vi "DAQ Viewer-Core_Process.vi"(0 "FTW Actor Instance Configuration":string="{\n  \"Identity\": \"ActorName\",\n  \"InboxAddress\": \"inproc://*\",\n  \"PublisherAddress\": \"\",\n  \"LoggerAddress\": \"\",\n  \"DebugEnableInboxLogging\": false,\n  \"DebugEnableJobLogging\": false,\n  \"LauncherAddress\": \"\",\n  \"My Data\": false\n}", 11 "ErrorIn":errorcluster) -> (15 "Error":errorcluster)   [LabVIEW 2013, in "DAQ Viewer-Core.lvclass"]
uses:
  DAQ Viewer-Core.lvclass
  source/actor/Message/Base/FTW-Message.lvclass
  source/actor/Instance/FTW-ActorInstance.lvclass/FTW-ActorInstance.ctl
  source/actor/JobSequencer/FTW-SEQ-Current.vi
  source/actor/Instance/FTW-ActorInstance.lvclass
  source/actor/Message/Request/FTW-Message-IncomingRequest.lvclass
panel:
  # "#TODO\nhide controls for a GUI"
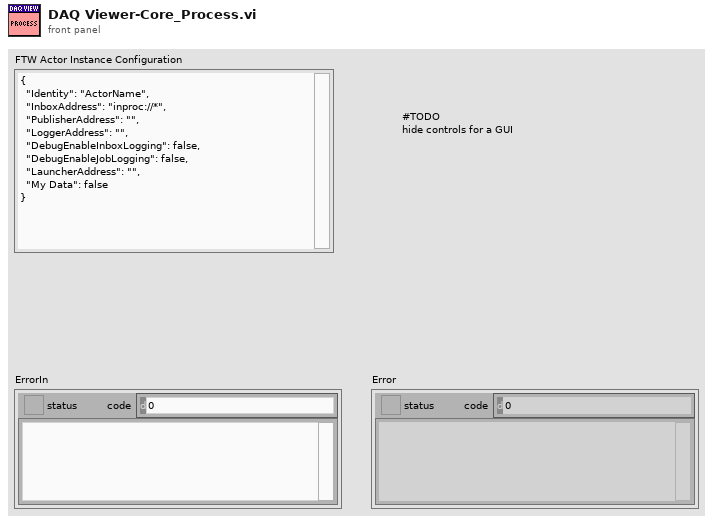
[diagram p1: front panel]
types:
  T1 = cluster{"Incoming Requests":refnum<event-registration>, "Local Messages":refnum<event-registration>, "Additional Registration Types":refnum<event-registration>}
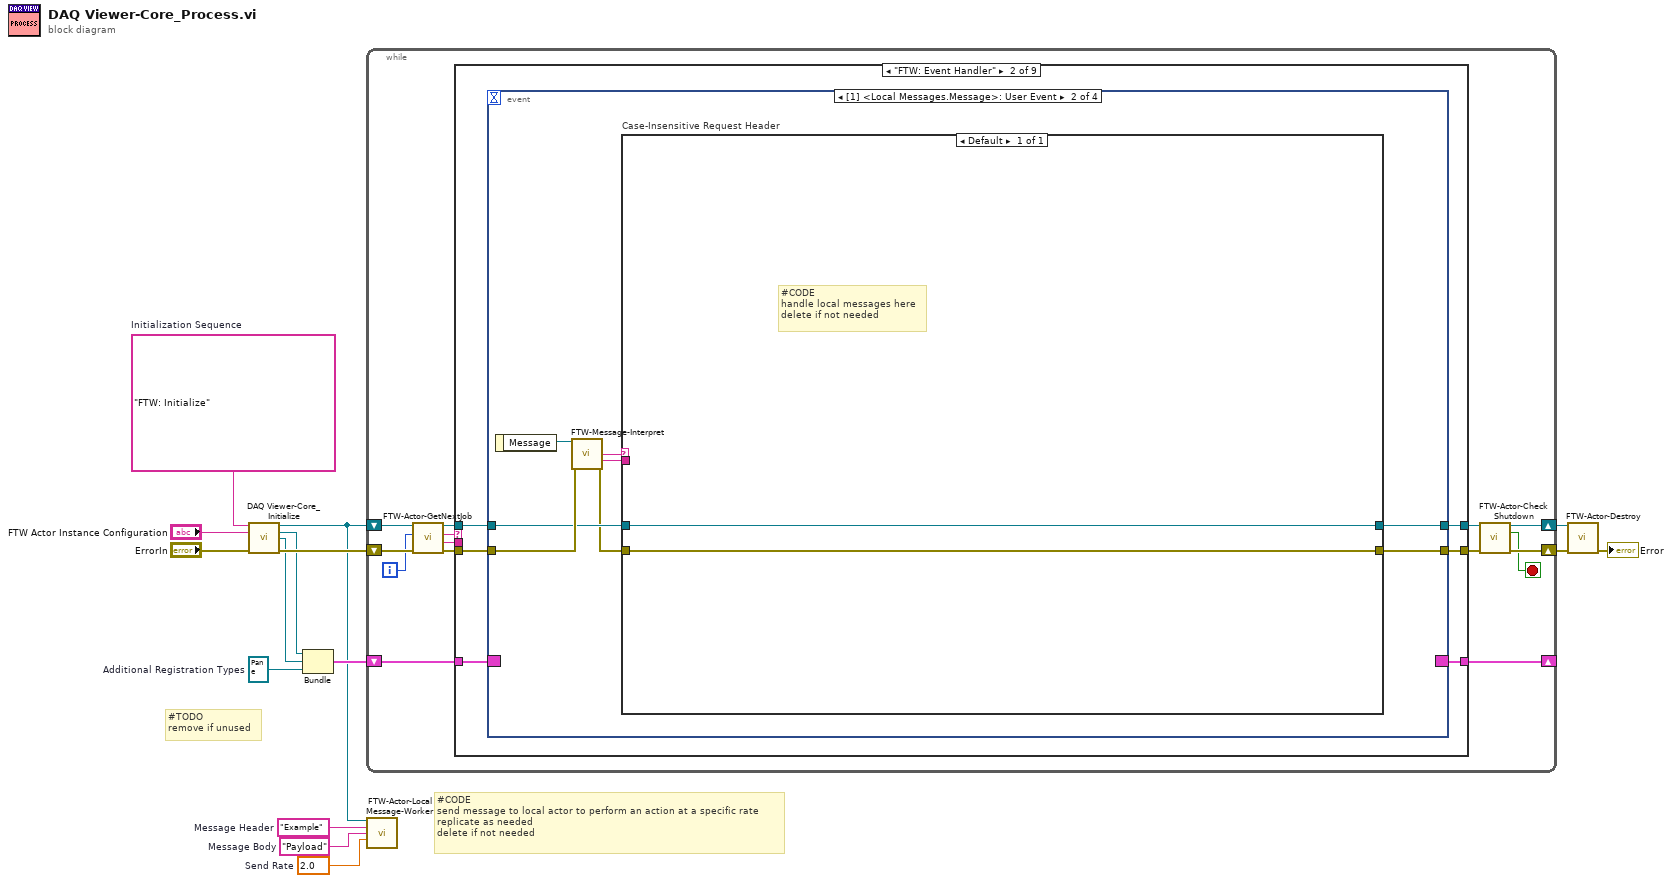
[diagram p0: block diagram]
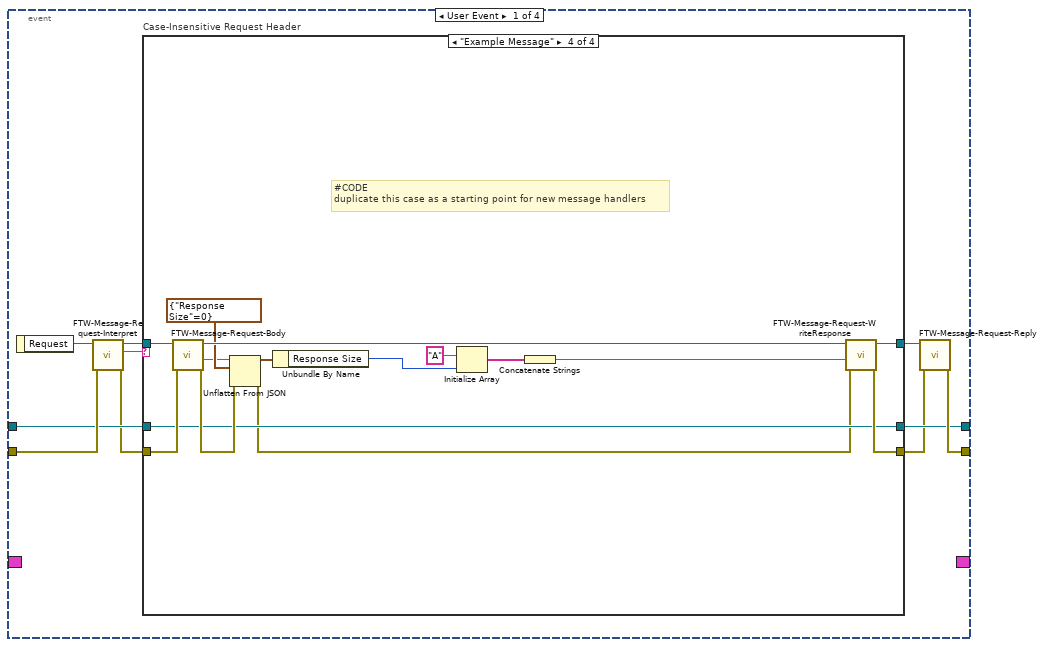
[diagram p3: hidden frame]
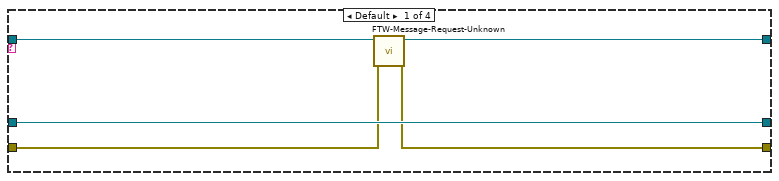
[diagram p4: hidden frame]
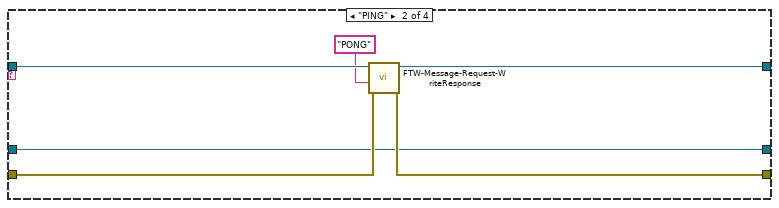
[diagram p5: hidden frame]
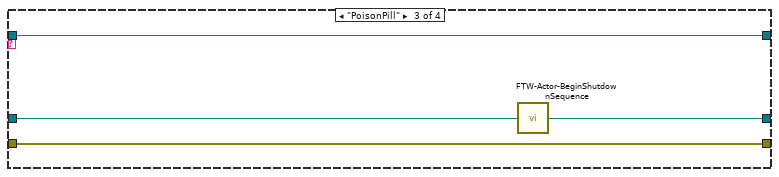
[diagram p6: hidden frame]
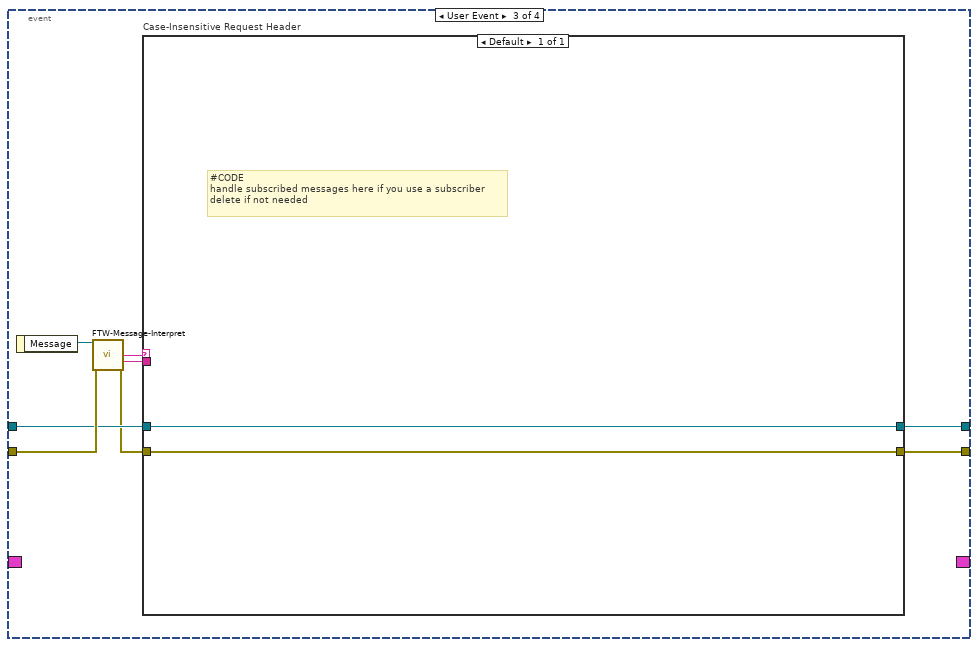
[diagram p7: hidden frame]
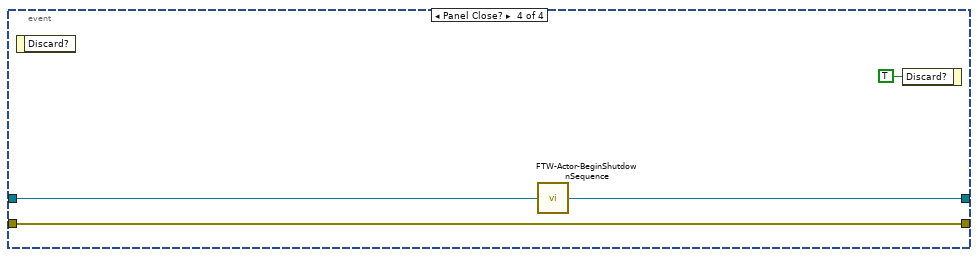
[diagram p8: hidden frame]
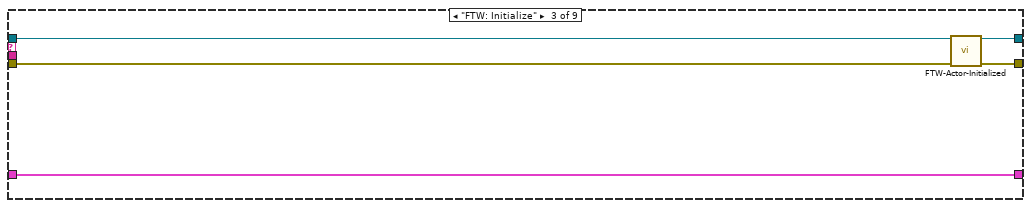
[diagram p9: hidden frame]
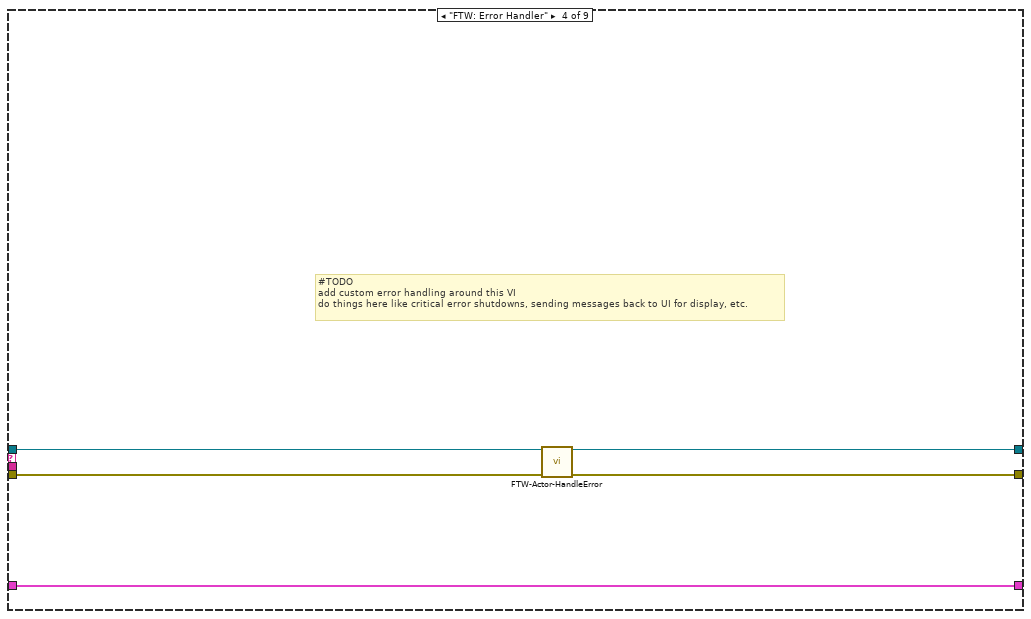
[diagram p10: hidden frame]
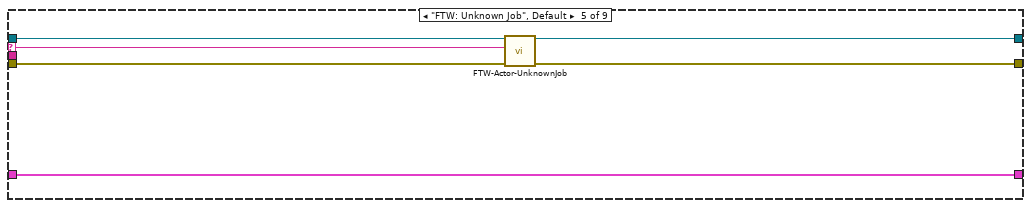
[diagram p11: hidden frame]
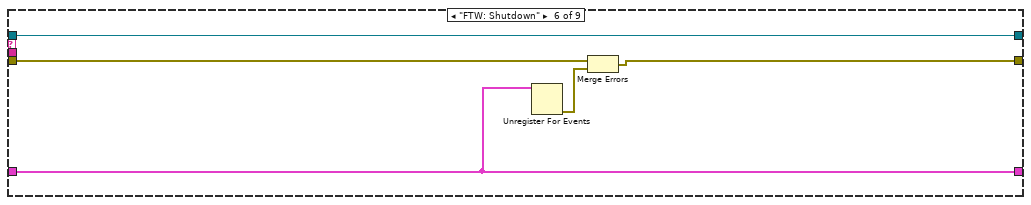
[diagram p12: hidden frame]
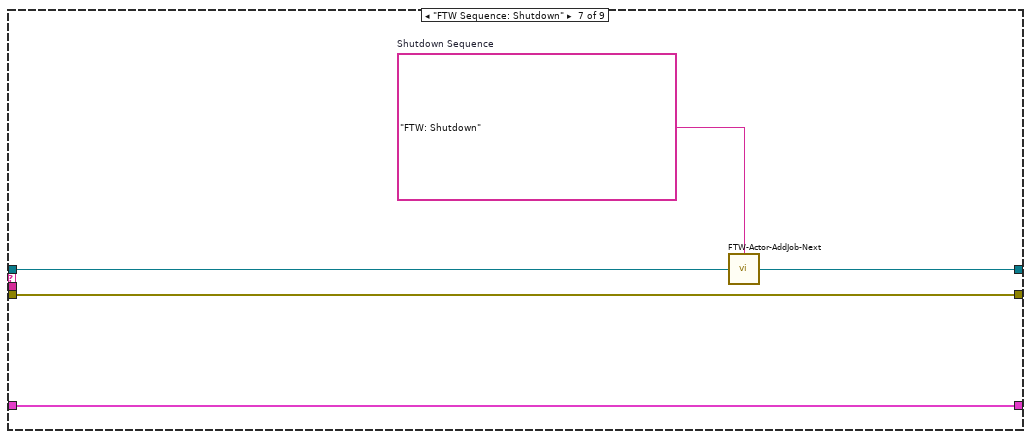
[diagram p13: hidden frame]
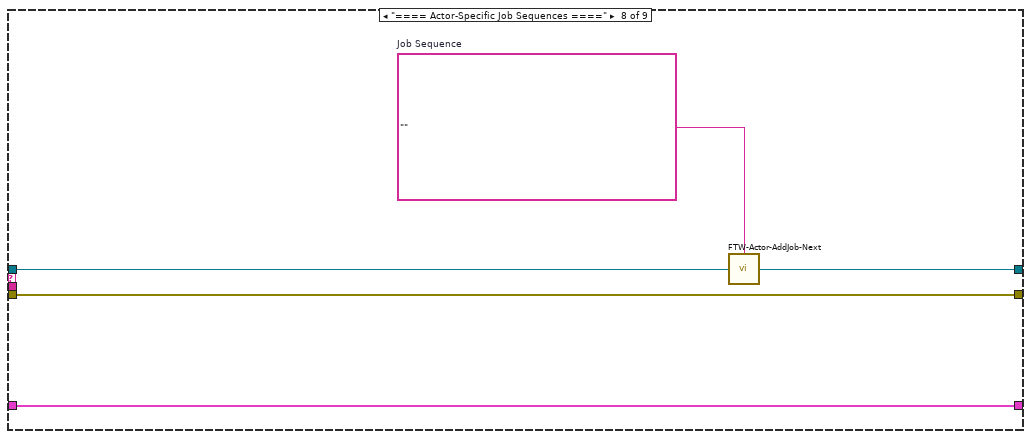
[diagram p14: hidden frame]
diagram:
  w2 = 2.0  # Send Rate
  w3 = "Payload"  # Message Body
  w4 = "Example"  # Message Header
  w5 = refnum<event-registration> refnum  # Additional Registration Types
  w11 = "FTW: Initialize"  # Initialization Sequence
  # "#CODE\nsend message to local actor to perform an action at a specific rate\nreplicate as needed\ndelete if not needed"
  # "#TODO\nremove if unused"
  n1 = call "DAQ Viewer-Core_Initialize.vi"("Initialization Sequence"=w11, "FTW Actor Instance Configuration"="FTW Actor Instance Configuration", "error in (no error)"="ErrorIn") -> ("Actor Template-Core out"=w1:refnum<class "DAQ Viewer-Core.lvclass">, "Incoming Requests"=w7:refnum<event-registration>, "Local Messages"=w6:refnum<event-registration>, "error out"=w12:errorcluster)  [unwired: 9 in]
  n2 = Bundle("Incoming Requests"=w7, "Local Messages"=w6, "Additional Registration Types"=w5) -> (w9:T1)  [unwired: 1 in]
  n3 = while {
    shift-right: [w19] -> w14
    shift-left: w12 -> [w26]
    shift-right: [w16] -> _
    shift-left: w9 -> [w29]
    shift-right: [w21] -> w15
    shift-left: w1 -> [w28]
    i -> [w17]
    stop <- w18 stop-if-true
    n4 = call "FTW-Actor-GetNextJob.vi"("error in"=w26, "Jobs Performed"=w17, "FTW Actor Instance"=w28) -> ("error out"=w25:errorcluster, "Job Data"=w23:string, "Job Name"=w24:string, "FTW Actor Instance out"=w27:refnum<class "DAQ Viewer-Core.lvclass">)  [unwired: 5 in]
    n5 = case shown="\"FTW: Event Handler\"" w24 {
      selector: w24 -> [_ _ _ _ w113 _ _ _ _]
      tunnel: [w31 w38 w103 w108 w116 w122 w127 w132 w136] -> w20
      tunnel: w25 -> [w31 w37 w106 w110 w117 w123 w127 w132 w136]
      tunnel: w29 -> [w32 w33 w107 w112 w118 w119 w128 w133 w135]
      tunnel: [w32 w36 w107 w112 w118 w119 w128 w133 w135] -> w16
      tunnel: w23 -> [_ _ _ _ _ _ _ _ _]
      tunnel: [w30 w35 w104 w109 w114 w120 w125 w130 w134] -> w22
      tunnel: w27 -> [w30 w34 w105 w111 w115 w120 w126 w131 w134]
      frame "==== Featherweight Framework Jobs ====" {
      }
      frame "FTW: Event Handler" {
        n6 = event shown="[1] <Local Messages.Message>: User Event" {
          selector: w33 -> [_ _ _ _]
          dyn-events: [_ _ _ _] -> w36
          timeout: _ -> [_ _ _ _]
          tunnel: [w47 w81 w91 w101] -> w38
          tunnel: w37 -> [w46 w85 w95 w101]
          tunnel: [w41 w82 w92 w99] -> w35
          tunnel: w34 -> [w45 w84 w94 w100]
          event User Event {
            n7 = event-data() -> ("Request"=w48:refnum<class "FTW-Message-IncomingRequest.lvclass">)  [unwired: 1 in]
            n8 = call "FTW-Message-Request-Interpret.vi"("error in"=w46, "FTW Incoming Request"=w48) -> ("error out"=w44:errorcluster, "Request Header"=w42:string, "FTW Incoming Request out"=w43:refnum<class "FTW-Message-IncomingRequest.lvclass">)  [unwired: 5 in, 2 out]
            n9 = case "Case-Insensitive Request Header" shown="\"Example Message\"" w42 {
              tunnel: [w51 w57 w62 w75] -> w40
              tunnel: w44 -> [w52 w58 w62 w78]
              tunnel: [w53 w56 w63 w72] -> w41
              tunnel: w45 -> [w53 w56 w61 w72]
              tunnel: w43 -> [w50 w59 w60 w76]
              tunnel: [w49 w55 w60 w73] -> w39
              frame Default {
                n10 = call "FTW-Message-Request-Unknown.vi"("error in"=w52, "FTW Incoming Request"=w50) -> ("error out"=w51:errorcluster, "FTW Incoming Request Out"=w49:refnum<class "FTW-Message-IncomingRequest.lvclass">)  [unwired: 8 in]
              }
              frame "PING" {
                n11 = call "FTW-Message-Request-WriteResponse.vi"("error in"=w58, "Response Body"="PONG" ("Response Header"), "FTW Incoming Request"=w59) -> ("error out"=w57:errorcluster, "FTW Incoming Request out"=w55:refnum<class "FTW-Message-IncomingRequest.lvclass">)  [unwired: 7 in]
              }
              frame "PoisonPill" {
                n12 = call "FTW-Actor-BeginShutdownSequence.vi"("FTW Actor Instance"=w61) -> ("FTW Actor Instance out"=w63:refnum<class "DAQ Viewer-Core.lvclass">)  [unwired: 3 in]
              }
              frame "Example Message" {
                # "#CODE\nduplicate this case as a starting point for new message handlers"
                n13 = call "FTW-Message-Request-Body.vi"("error in"=w78, "FTW Incoming Request"=w76) -> ("error out"=w77:errorcluster, "Request Body"=w69:string, "FTW Incoming Request out"=w74:refnum<class "FTW-Message-IncomingRequest.lvclass">)  [unwired: 7 in]
                n14 = Unflatten From JSON(JSON string=w69, type and defaults=cluster{"Response Size":i32} {"Response Size"=0}, error in (no error)=w77) -> (value=w68:cluster{"Response Size":i32}, error out=w71:errorcluster)  [unwired: 4 in]
                n15 = Unbundle By Name(w68) -> ("Response Size"=w67:i32)
                n16 = Initialize Array("A", w67) -> (w65:string[])
                n17 = Concatenate Strings(w65) -> (w64:string)
                n18 = call "FTW-Message-Request-WriteResponse.vi"("error in"=w71, "Response Body"=w64, "FTW Incoming Request"=w74) -> ("error out"=w75:errorcluster, "FTW Incoming Request out"=w73:refnum<class "FTW-Message-IncomingRequest.lvclass">)  [unwired: 7 in]
              }
            }
            n19 = call "FTW-Message-Request-Reply.vi"("FTW: Reply Error"=w40, "FTW Incoming Request"=w39) -> ("error out"=w47:errorcluster)  [unwired: 8 in, 1 out]
          }
          event User Event {
            n20 = event-data() -> ("Message"=w86:refnum<class "FTW-Message.lvclass">)  [unwired: 1 in]
            n21 = call-dynamic "FTW-Message-Interpret.vi"("FTW Message"=w86, "error in"=w85) -> ("Message Header"=w80:string, "Message Body"=w79:string, "error out"=w83:errorcluster)  [unwired: 9 in, 2 out]
            n22 = case "Case-Insensitive Request Header" shown="Default" w80 {
              tunnel: [w87] -> w81
              tunnel: w83 -> [w87]
              tunnel: [w88] -> w82
              tunnel: w84 -> [w88]
              tunnel: w79 -> [_]
              frame Default {
                # "#CODE\nhandle local messages here\ndelete if not needed"
              }
            }
          }
          event User Event {
            n23 = event-data() -> ("Message"=w96:refnum<class "FTW-Message.lvclass">)  [unwired: 1 in]
            n24 = call-dynamic "FTW-Message-Interpret.vi"("FTW Message"=w96, "error in"=w95) -> ("Message Header"=w90:string, "Message Body"=w89:string, "error out"=w93:errorcluster)  [unwired: 9 in, 2 out]
            n25 = case "Case-Insensitive Request Header" shown="Default" w90 {
              tunnel: [w97] -> w91
              tunnel: w93 -> [w97]
              tunnel: [w98] -> w92
              tunnel: w94 -> [w98]
              tunnel: w89 -> [_]
              frame Default {
                # "#CODE\nhandle subscribed messages here if you use a subscriber\ndelete if not needed"
              }
            }
          }
          event Panel Close? {
            n26 = event-data() -> ()  [unwired: 1 in, 1 out]
            n27 = call "FTW-Actor-BeginShutdownSequence.vi"("FTW Actor Instance"=w100) -> ("FTW Actor Instance out"=w99:refnum<class "DAQ Viewer-Core.lvclass">)  [unwired: 3 in]
            n28 = event-data("Discard?"=TRUE) -> ()  [unwired: 1 in, 1 out]
          }
        }
      }
      frame "FTW: Initialize" {
        n29 = call-dynamic "FTW-Actor-Initialized.vi"("FTW Actor Instance"=w105, "error in"=w106) -> ("FTW Actor Instance out"=w104:refnum<class "DAQ Viewer-Core.lvclass">, "error out"=w103:errorcluster)  [unwired: 12 in]
      }
      frame "FTW: Error Handler" {
        # "#TODO\nadd custom error handling around this VI\ndo things here like critical error shutdowns, sending messages back to UI for display, etc."
        n30 = call-dynamic "FTW-Actor-HandleError.vi"("FTW Actor Instance"=w111, "error in"=w110) -> ("FTW Actor Instance out"=w109:refnum<class "DAQ Viewer-Core.lvclass">, "error out"=w108:errorcluster)  [unwired: 10 in, 2 out]
      }
      frame "FTW: Unknown Job", Default {
        n31 = call-dynamic "FTW-Actor-UnknownJob.vi"("FTW Actor Instance"=w115, "Unknown Job"=w113, "error in"=w117) -> ("FTW Actor Instance out"=w114:refnum<class "DAQ Viewer-Core.lvclass">, "error out"=w116:errorcluster)  [unwired: 11 in]
      }
      frame "FTW: Shutdown" {
        n32 = Unregister For Events(event registration refnum=w119) -> (error out=w121:errorcluster)  [unwired: 1 in]
        n33 = Merge Errors(w123, w121) -> (w122:errorcluster)
      }
      frame "FTW Sequence: Shutdown" {
        w124 = "FTW: Shutdown"  # Shutdown Sequence
        n34 = call "FTW-Actor-AddJob-Next.vi"("Add Next in Job Queue"=w124, "FTW Actor Instance"=w126) -> ("FTW Actor Instance out"=w125:refnum<class "DAQ Viewer-Core.lvclass">)  [unwired: 2 in]
      }
      frame "==== Actor-Specific Job Sequences ====" {
        w129 = ""  # Job Sequence
        n35 = call "FTW-Actor-AddJob-Next.vi"("Add Next in Job Queue"=w129, "FTW Actor Instance"=w131) -> ("FTW Actor Instance out"=w130:refnum<class "DAQ Viewer-Core.lvclass">)  [unwired: 2 in]
      }
      frame "==== Actor-Specific Jobs ====" {
      }
    }
    n36 = call "FTW-Actor-CheckShutdown.vi"("FTW Actor Instance"=w22, "error in"=w20) -> ("FTW Actor Instance out"=w21:refnum<class "DAQ Viewer-Core.lvclass">, "Shutdown?"=w18:bool, "error out"=w19:errorcluster)  [unwired: 11 in]
  }
  n37 = call-dynamic "FTW-Actor-LocalMessage-Worker.vi"("FTW-ActorInstance In"=w1, "Message Header"=w4, "Message Body"=w3, "Send Rate"=w2) -> ()  [unwired: 12 in]
  n38 = call-dynamic "FTW-Actor-Destroy.vi"("FTW Actor Instance"=w15, "error in"=w14) -> ("error out"=→"Error":errorcluster)  [unwired: 13 in]
